vi "Read Current Peak Limits.vi"(0 "VISA resource name":refnum<visa-resource-name>, 11 "error in (no error)":errorcluster) -> (4 "VISA resource name out":refnum<visa-resource-name>, 6 "Current Peak Low Limit (A)":dbl, 8 "Current Peak High Limit (A)":dbl, 15 "error out":errorcluster)   [LabVIEW 2014, in "eec 6700.lvlib"]
doc: "Reads the Current Peak limits set in the active step of the power source instrument.\n\nNote : This VI should be used i program mode"
uses:
  <instrlib>/eec 6700/eec 6700.lvlib
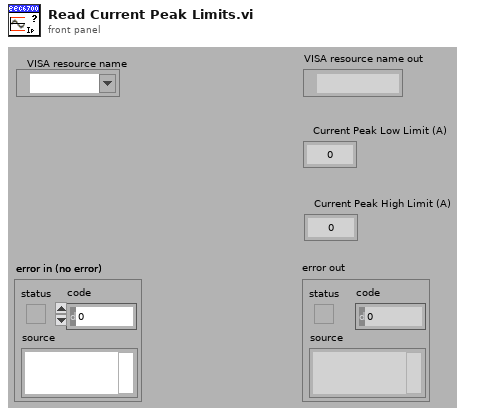
[diagram p1: front panel]
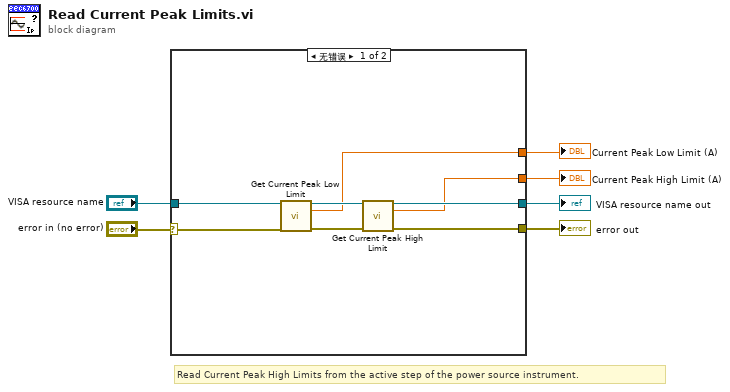
[diagram p0: block diagram]
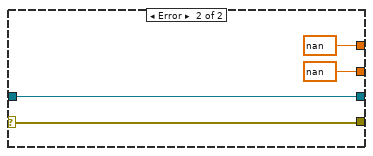
[diagram p2: hidden frame]
diagram:
  # "Read Current Peak High Limits from the active step of the power source instrument."
  n1 = case shown="无错误" "error in (no error)" {
    selector: "error in (no error)" -> [w14 w15]
    tunnel: [w12 w15] -> w5
    tunnel: [w11 w16] -> w4
    tunnel: "VISA resource name" -> [w9 w16]
    tunnel: [w7 nan ("Voltage Low Limit")] -> w2
    tunnel: [w8 nan ("Voltage Low Limit")] -> w1
    frame No Error {
      n2 = call <instrlib>:"Get Current Peak Low Limit.vi"("VISA resource name"=w9, "error in (no error)"=w14) -> ("VISA resource name out"=w10:refnum<visa-resource-name>, "Current Peak Low Limit (A)"=w7:dbl, "error out"=w13:errorcluster)  [unwired: 11 in]
      n3 = call <instrlib>:"Get Current Peak High Limit.vi"("VISA resource name"=w10, "error in (no error)"=w13) -> ("VISA resource name out"=w11:refnum<visa-resource-name>, "Current Peak High Limit (A)"=w8:dbl, "error out"=w12:errorcluster)  [unwired: 11 in]
    }
    frame Error {
    }
  }
  "error out" <- w5
  "VISA resource name out" <- w4
  "Current Peak High Limit (A)" <- w1
  "Current Peak Low Limit (A)" <- w2
